vi "AutomatedBeamGage_ManualStepTable.vi"() -> ()   [LabVIEW 2016]
uses:
  C:/Program Files/Spiricon/BeamSquared/M2.Automation.dll
  M2.Automation.dll
panel:
  out "RunStatus":i32(ring) items=["READY", "RUNNING", "RUN_FINISHED", "UNAVAILABLE", "ABORTED", "LOADING", "ERROR"]
  in  "Save Run Settings":bool
  in  "Shutdown Server":bool
  in  "ManualStepArray":dbl[](array[numeric])
  in  "Save Step Table":bool
  in  "Start/Stop Run":bool
  out "FrameAnalyzerStatus":i32
  in  "Model":string
  in  "Comment":string
  in  "CorrectForSmear":bool
  in  "FittedDivergence":bool
  in  "LaserLocation":dbl
  in  "FocalLength":dbl
  in  "WaveLength":dbl
  in  "SerialNumber":string
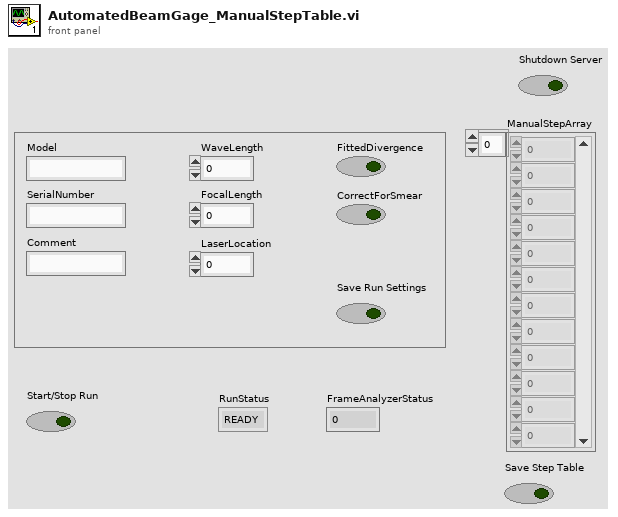
[diagram p1: front panel]
types:
  T1 = cluster{"AAnalyzerStatus":i32, "ARunManagerStatus":i32}
  T2 = cluster{"notifier out":refnum<notifier>, "new reference":refnum<k24>}
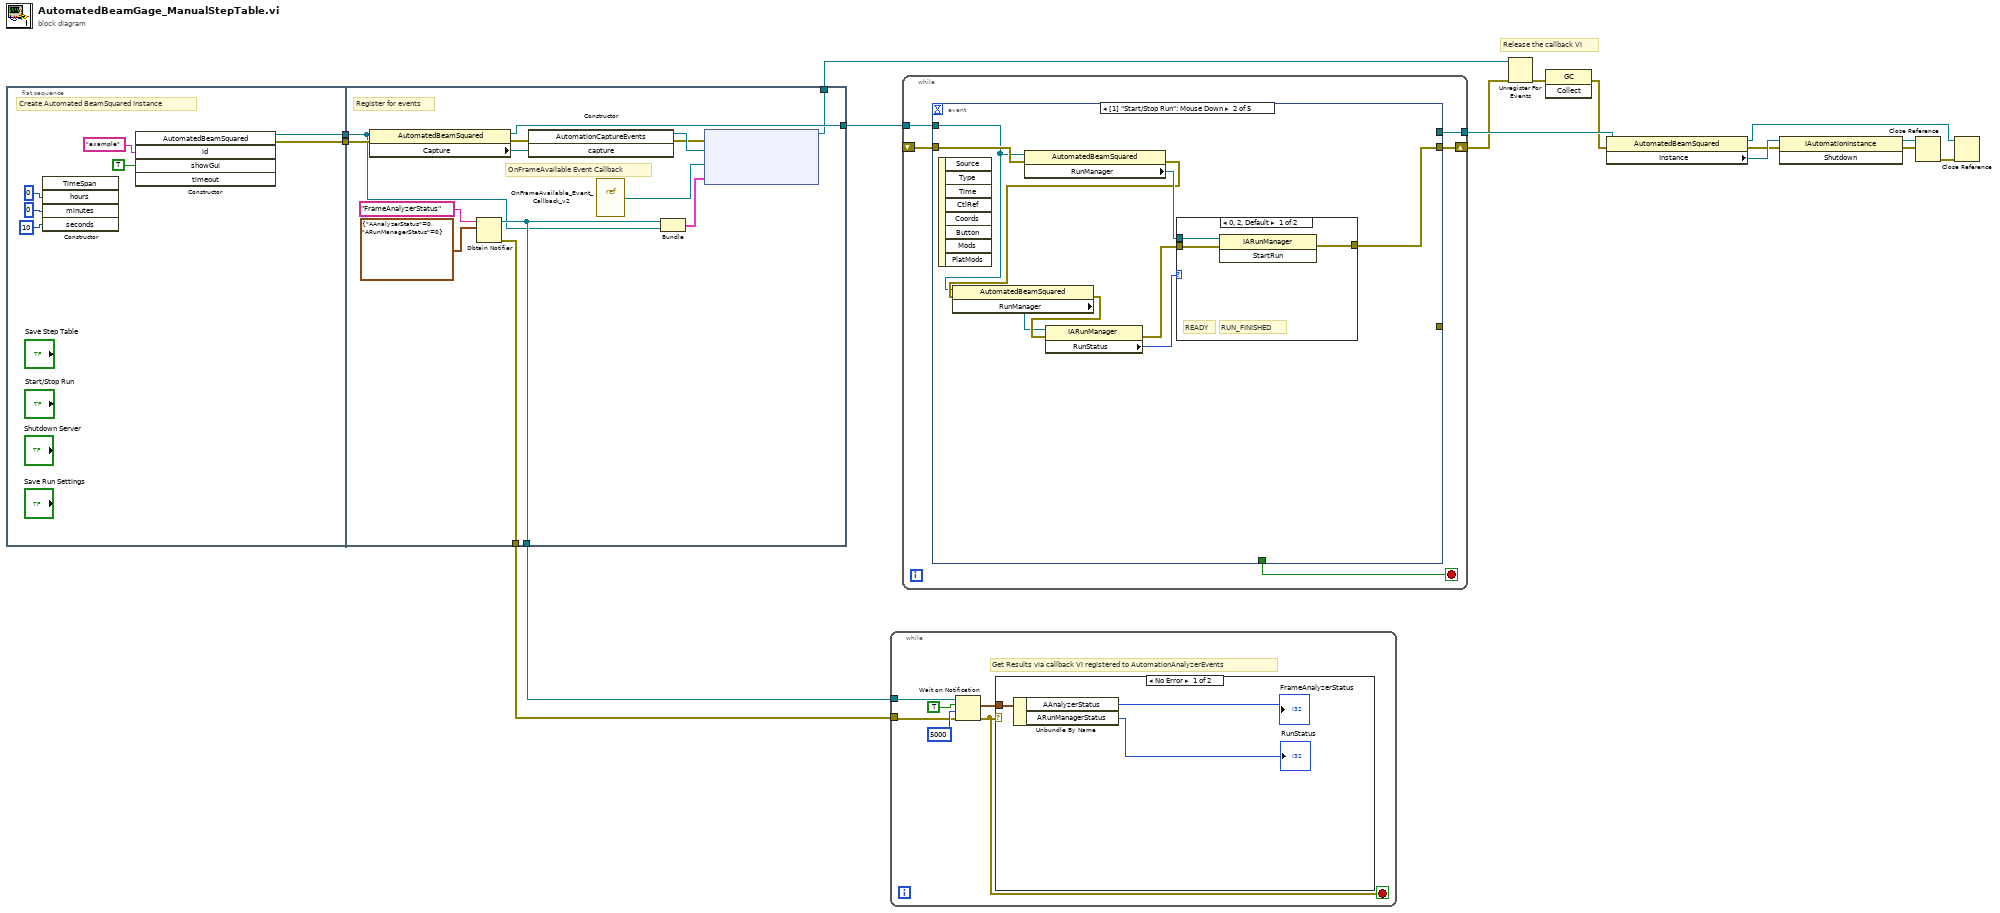
[diagram p0: block diagram]
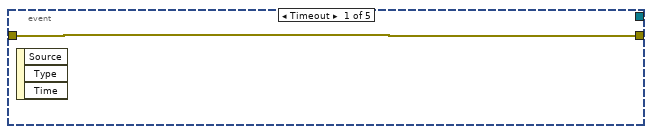
[diagram p3: hidden frame]
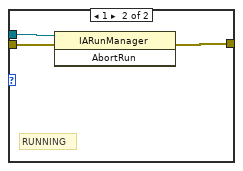
[diagram p4: hidden frame]
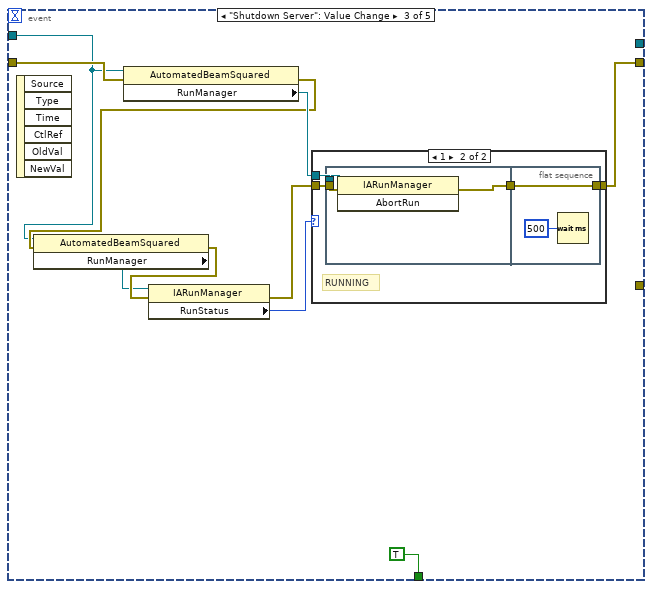
[diagram p5: hidden frame]
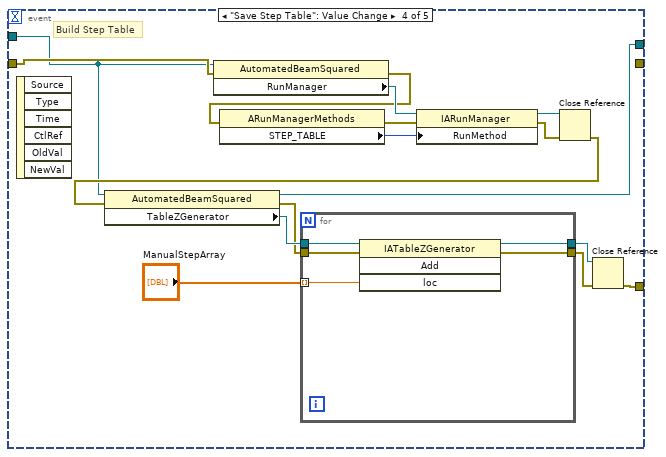
[diagram p7: hidden frame]
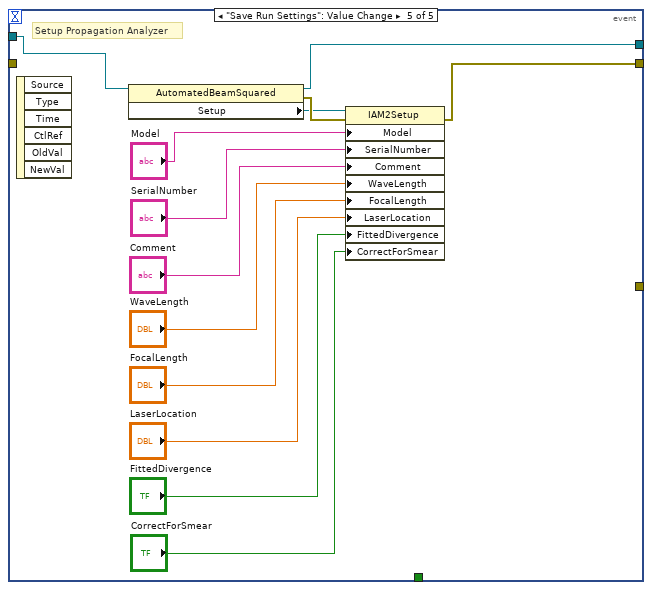
[diagram p8: hidden frame]
diagram:
  # "Release the callback VI"
  n1 = flat-sequence {
    tunnel: [w18] -> w16
    tunnel: [w17] -> w15
    tunnel: [w28] -> w8
    tunnel: w15 -> [w25]
    tunnel: w16 -> [w31]
    tunnel: [w27] -> w4
    tunnel: [w26] -> w6
    tunnel: [w24] -> w3
    frame #0 {
      # "Create Automated BeamSquared Instance"
      n2 = constructor class="TimeSpan"("hours"=0, "minutes"=0, "seconds"=10) -> ()  [unwired: 3 in, 6 out]
      n3 = constructor class="AutomatedBeamSquared"("id"="example", "showGui"=TRUE) -> (reference out=w17:refnum<k24>, error out=w18:errorcluster)  [unwired: 4 in, 4 out]
    }
    frame #1 {
      # "OnFrameAvailable Event Callback"
      # "Register for events"
      n4 = property class="AutomatedBeamSquared"(reference=w25, error in=w31) -> (reference out=w26:refnum<k24>, error out=w30:errorcluster, "Capture"=w32:refnum<k24>)
      n5 = Obtain Notifier(name (unnamed)="FrameAnalyzerStatus", notification data type=T1 {"AAnalyzerStatus"=0, "ARunManagerStatus"=0}) -> (notifier out=w27:refnum<notifier>, error out=w28:errorcluster)  [unwired: 2 in, 1 out]
      n6 = constructor class="AutomationCaptureEvents"(error in=w30, "capture"=w32) -> (reference out=w37:refnum<k24>, error out=w36:errorcluster)  [unwired: 2 in, 2 out]
      n7 = vi-ref "OnFrameAvailable_Event_Callback_v2.vi"() -> ("vi reference"=w34:refnum<vi>)
      n8 = Bundle("notifier out"=w27, "new reference"=w25) -> (w29:T2)  [unwired: 1 in]
      n9 = node(w36, w37, w34, w29) -> (w24:refnum<k27>)  [unwired: 1 in, 1 out]
    }
  }
  n10 = while {
    tunnel: w8 -> [w41]
    tunnel: w4 -> [w38]
    stop <- w39 stop-if-true
    # "Get Results via callback VI registered to AutomationAnalyzerEvents"
    n11 = Wait on Notification(notifier=w38, ignore previous (F)=TRUE, timeout in ms (-1)=5000, error in (no error)=w41) -> (notification=w40:T1, error out=w39:errorcluster)  [unwired: 2 out]
    n12 = case shown="No Error" w39 {
      tunnel: w40 -> [w46 _]
      frame No Error {
        n13 = Unbundle By Name(w46) -> ("AAnalyzerStatus"=→"FrameAnalyzerStatus":i32, "ARunManagerStatus"=→"RunStatus":i32)
      }
      frame Error {
      }
    }
  }
  n14 = while {
    shift-right: [w50] -> w5
    shift-left: _ -> [w51]
    tunnel: [w48] -> w7
    tunnel: w6 -> [w47]
    stop <- w49 stop-if-true
    n15 = event shown="[1] \"Start/Stop Run\": Mouse Down" {
      selector: _ -> [_ _ _ _ _]
      dyn-events: _ -> [_ _ _ _ _]
      timeout: _ -> [_ _ _ _ _]
      tunnel: w51 -> [w52 w61 w77 w93 _]
      tunnel: [w52 w54 w70 _ w109] -> w50
      tunnel: [_ _ TRUE _ _] -> w49
      tunnel: [_ _ _ w100 _] -> _
      tunnel: [_ _ _ w89 w110] -> w48
      tunnel: w47 -> [_ w53 w68 w88 w111]
      event Timeout {
        n16 = event-data() -> ()  [unwired: 1 in, 3 out]
      }
      event "Start/Stop Run": Mouse Down {
        n17 = event-data() -> ()  [unwired: 1 in, 8 out]
        n18 = property class="AutomatedBeamSquared"(reference=w53, error in=w61) -> (error out=w58:errorcluster, "RunManager"=w60:refnum<k24>)  [unwired: 1 out]
        n19 = property class="AutomatedBeamSquared"(reference=w53, error in=w58) -> (error out=w59:errorcluster, "RunManager"=w57:refnum<k24>)  [unwired: 1 out]
        n20 = property class="IARunManager"(reference=w57, error in=w59) -> (error out=w55:errorcluster, "RunStatus"=w56:i32)  [unwired: 1 out]
        n21 = case shown="0, 2, Default" w56 {
          tunnel: w60 -> [w64 w67]
          tunnel: w55 -> [w63 w66]
          tunnel: [w62 w65] -> w54
          frame 0, 2, Default {
            # "RUN_FINISHED"
            # "READY"
            n22 = invoke class="IARunManager" method="StartRun"(reference=w64, error in=w63) -> (error out=w62:errorcluster)  [unwired: 1 in, 2 out]
          }
          frame 1 {
            # "RUNNING"
            n23 = invoke class="IARunManager" method="AbortRun"(reference=w67, error in=w66) -> (error out=w65:errorcluster)  [unwired: 1 in, 2 out]
          }
        }
      }
      event "Shutdown Server": Value Change {
        n24 = event-data() -> ()  [unwired: 1 in, 6 out]
        n25 = property class="AutomatedBeamSquared"(reference=w68, error in=w77) -> (error out=w74:errorcluster, "RunManager"=w76:refnum<k24>)  [unwired: 1 out]
        n26 = property class="AutomatedBeamSquared"(reference=w68, error in=w74) -> (error out=w75:errorcluster, "RunManager"=w73:refnum<k24>)  [unwired: 1 out]
        n27 = property class="IARunManager"(reference=w73, error in=w75) -> (error out=w71:errorcluster, "RunStatus"=w72:i32)  [unwired: 1 out]
        n28 = case shown="1" w72 {
          tunnel: w76 -> [_ w82]
          tunnel: w71 -> [w78 w81]
          tunnel: [w78 w80] -> w70
          frame 0, 2, Default {
            # "RUN_FINISHED"
            # "READY"
          }
          frame 1 {
            # "RUNNING"
            n29 = flat-sequence {
              tunnel: w82 -> [w85]
              tunnel: w81 -> [w84]
              tunnel: [w83] -> w79
              tunnel: [w87] -> w80
              tunnel: w79 -> [w87]
              frame #0 {
                n30 = invoke class="IARunManager" method="AbortRun"(reference=w85, error in=w84) -> (error out=w83:errorcluster)  [unwired: 1 in, 2 out]
              }
              frame #1 {
                n31 = Wait (ms)(milliseconds to wait=u32 500) -> ()  [unwired: 1 out]
              }
            }
          }
        }
      }
      event "Save Step Table": Value Change {
        # "Build Step Table"
        n32 = event-data() -> ()  [unwired: 1 in, 6 out]
        n33 = property class="AutomatedBeamSquared"(reference=w88, error in=w93) -> (error out=w95:errorcluster, "RunManager"=w97:refnum<k24>)  [unwired: 1 out]
        n34 = property class="ARunManagerMethods"(error in=w95) -> (error out=w96:errorcluster, "STEP_TABLE"=w94:i32)  [unwired: 1 in, 1 out]
        n35 = property class="IARunManager"(reference=w97, error in=w96, "RunMethod"=w94) -> (reference out=w98:refnum<k24>, error out=w99:errorcluster)
        n36 = Close Reference(reference=w98, error in (no error)=w99) -> (error out=w90:errorcluster)
        n37 = property class="AutomatedBeamSquared"(reference=w88, error in=w90) -> (reference out=w89:refnum<k24>, error out=w102:errorcluster, "TableZGenerator"=w103:refnum<k24>)
        n38 = for {
          tunnel: "ManualStepArray" -> [w108] mode=indexing
          tunnel: w102 -> [w107]
          tunnel: [w106] -> w92
          tunnel: [w105] -> w91
          tunnel: w103 -> [w104]
          n39 = invoke class="IATableZGenerator" method="Add"(reference=w104, error in=w107, "loc"=w108) -> (reference out=w105:refnum<k24>, error out=w106:errorcluster)  [unwired: 1 in, 2 out]
        }
        n40 = Close Reference(reference=w91, error in (no error)=w92) -> (error out=w100:errorcluster)
      }
      event "Save Run Settings": Value Change {
        # "Setup Propagation Analyzer"
        n41 = event-data() -> ()  [unwired: 1 in, 6 out]
        n42 = property class="AutomatedBeamSquared"(reference=w111) -> (reference out=w110:refnum<k24>, error out=w113:errorcluster, "Setup"=w112:refnum<k24>)  [unwired: 1 in]
        n43 = property class="IAM2Setup"(reference=w112, error in=w113, "Model"="Model", "SerialNumber"="SerialNumber", "Comment"="Comment", "WaveLength"="WaveLength", "FocalLength"="FocalLength", "LaserLocation"="LaserLocation", "FittedDivergence"="FittedDivergence", "CorrectForSmear"="CorrectForSmear") -> (error out=w109:errorcluster)  [unwired: 1 out]
      }
    }
  }
  n44 = Unregister For Events(event registration refnum=w3, error in=w5) -> (error out=w2:errorcluster)
  n45 = invoke class="GC" method="Collect"(error in=w2) -> (error out=w1:errorcluster)  [unwired: 2 in, 2 out]
  n46 = property class="AutomatedBeamSquared"(reference=w7, error in=w1) -> (reference out=w11:refnum<k24>, error out=w9:errorcluster, "Instance"=w10:refnum<k24>)
  n47 = invoke class="IAutomationInstance" method="Shutdown"(reference=w10, error in=w9) -> (reference out=w12:refnum<k24>, error out=w13:errorcluster)  [unwired: 1 in, 1 out]
  n48 = Close Reference(reference=w12, error in (no error)=w13) -> (error out=w14:errorcluster)
  n49 = Close Reference(reference=w11, error in (no error)=w14) -> ()  [unwired: 1 out]
